vi "AlliGator Visible Tab Label.vi"(8 "Error In":errorcluster) -> (0 "Error Out":errorcluster, 3 "Visible Tab":string)   [LabVIEW 2021, in "AlliGator Globals, Variables & Constants.lvlib"]
doc: "Returns the label of visible tab on AlliGator's main window."
uses:
  AlliGator Globals, Variables & Constants.lvlib
  AlliGator Refnums List.ctl
panel:
  # "see the AlliGator License on the block diagram (Ctrl+E or Window:Show Block Diagram)"
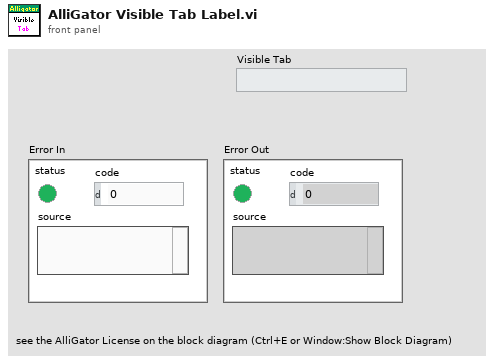
[diagram p1: front panel]
types:
  T1 = typedef "AlliGator Globals, Variables & Constants.lvlib/AlliGator Refnums List.ctl" = enum16{"---------- AlliGator Controls ----------", "AlliGator Tab Control Refnum", "---------- AlliGator Indicators ----------", "Source Image Display Refnum", "Phasor Plot Display Refnum", "Decay Fit Parameter Map Refnum", "---------- AlliGator VIs ----------", "AlliGator Settings Refnum", "AlliGator Launcher Refnum"}
  T2 = enum32{"Image Histogram", "Fluorescence Decay", "Fluorescence Decay Statistics", "Intensity Time Trace", "Phasor Plot", "Phasor Graph", "Phasor Ratio", "Lifetime & Other Parameters", "Decay Fit Parameter Map"}
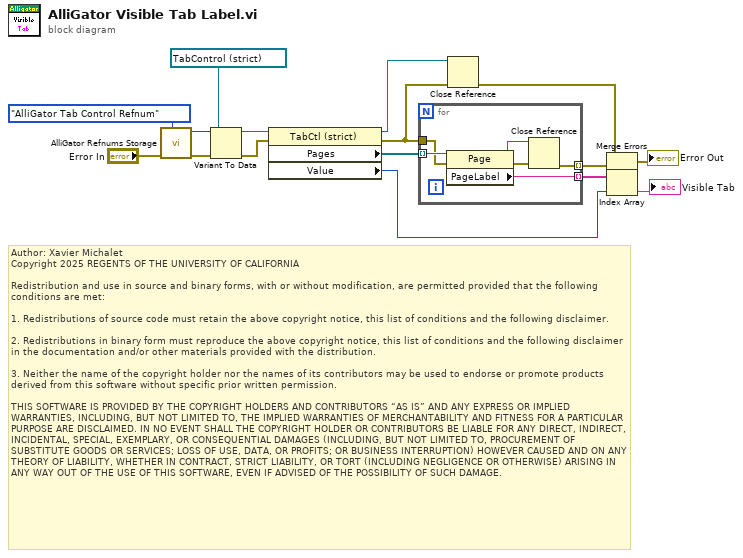
[diagram p0: block diagram]
diagram:
  # "Author: Xavier Michalet\nCopyright 2025 REGENTS OF THE UNIVERSITY OF CALIFORNIA\n\nRedistribution and use in source and binary forms, with or without modification, are permitted provided that the following conditions are met:\n\n1. Redistributions of source code must retain the above copyright notice, this list of conditions and the following disclaimer.\n\n2. Redistributions in binary form must reproduce the above copyright notice, this list of conditions and the following disclaimer in the documentation and/or other materials provided with the distribution.\n\n3. Neither the name of the copyright holder nor the names of its contributors may be used to endorse or promote products derived from this software without specific prior written permission.\n\nTHIS SOFTWARE IS PROVIDED BY THE COPYRIGHT HOLDERS AND CONTRIBUTORS “AS IS” AND ANY EXPRESS OR IMPLIED WARRANTIES, INCLUDING, BUT NOT LIMITED TO, THE IMPLIED WARRANTIES OF MERCHANTABILITY AND FITNESS FOR A PARTICULAR PURPOSE ARE DISCLAIMED. IN NO EVENT SHALL THE COPYRIGHT HOLDER OR CONTRIBUTORS BE LIABLE FOR ANY DIRECT, INDIRECT, INCIDENTAL, SPECIAL, EXEMPLARY, OR CONSEQUENTIAL DAMAGES (INCLUDING, BUT NOT LIMITED TO, PROCUREMENT OF SUBSTITUTE GOODS OR SERVICES; LOSS OF USE, DATA, OR PROFITS; OR BUSINESS INTERRUPTION) HOWEVER CAUSED AND ON ANY THEORY OF LIABILITY, WHETHER IN CONTRACT, STRICT LIABILITY, OR TORT (INCLUDING NEGLIGENCE OR OTHERWISE) ARISING IN ANY WAY OUT OF THE USE OF THIS SOFTWARE, EVEN IF ADVISED OF THE POSSIBILITY OF SUCH DAMAGE."
  n1 = call "AlliGator Refnums Storage.vi"("AlliGator Refnum List"=AlliGator_Refnums_List."AlliGator Tab Control Refnum", "Error In"="Error In") -> ("Error Out"=w7:errorcluster, "Data out"=w6:variant)  [unwired: 8 in]
  n2 = Variant To Data(error in=w7, type=refnum<vi> refnum ("AlliGator Tab Control Refnum"), Variant=w6) -> (data=w4:refnum<vi>, error out=w2:errorcluster)
  n3 = property class="TabCtl (strict)"(reference=w4, error in=w2) -> (reference out=w15:refnum<vi>, error out=w13:errorcluster, "Pages"=w16:refnum<vi>[], "Value"=w8:T2)
  n4 = for {
    tunnel: w16 -> [w22] mode=indexing
    tunnel: [w21] -> w14 mode=indexing
    tunnel: w13 -> [w20]
    tunnel: [w17] -> w12 mode=indexing
    n5 = property class="Page"(reference=w22, error in=w20) -> (reference out=w19:refnum<vi>, error out=w18:errorcluster, "PageLabel"=w21:string)
    n6 = Close Reference(reference=w19, error in (no error)=w18) -> (error out=w17:errorcluster)
  }
  n7 = Close Reference(reference=w15, error in (no error)=w13) -> (error out=w10:errorcluster)
  n8 = Merge Errors(w10, w12) -> (→"Error Out":errorcluster)
  n9 = Index Array(array=w14, index=w8) -> (element=→"Visible Tab":string)
